vi "이벤트 키 입력 예제.vi"() -> ()   [LabVIEW 2025]
panel:
  out "Boolean":bool
  out "key":string
  in  "stop":bool
  out "count":i32
  # "실행하면 키 입력값을 받고 엔터를 누르면 버튼에 불이 들어오는 구조"
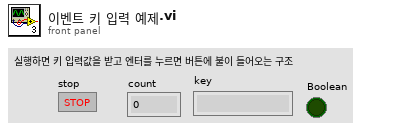
[diagram p1: front panel]
types:
  T1 = typedef "eventvkey.ctl" = enum16{"ASCII", "Enter", "Return", "Shift", "Ctrl", "Alt", "Cmd", "Opt", "Caps", "NumLock", "Clear", "Break", "Up", "Down", "Left", "Right", "Insert", "Delete", "Home", "End", "PageUp", "PageDown", "Escape", "Help", "Pause", "ScrollLock", "F1", "F2", "F3", "F4", "F5", "F6", "F7", "F8", "F9", "F10", "F11", "F12", "F13", "F14", "F15", "F16", "F17", "F18", "F19", "F20", "F21", "F22", "F23", "F24", "Play", "VolumeUp", "VolumeDown", "Mute", "Two Byte Char"}
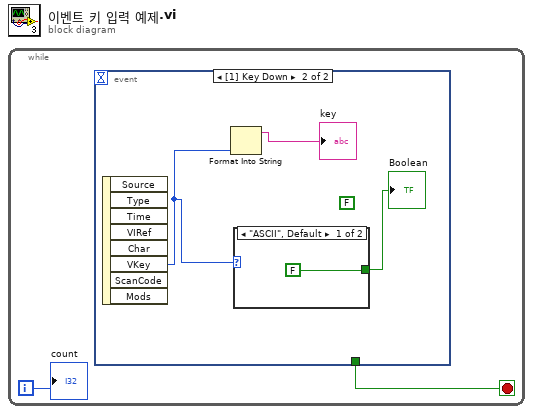
[diagram p0: block diagram]
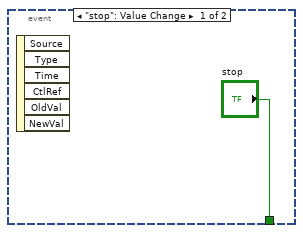
[diagram p2: hidden frame]
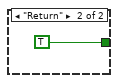
[diagram p3: hidden frame]
diagram:
  n1 = while {
    i -> [w2]
    stop <- w1 stop-if-true
    n2 = event shown="[1] Key Down" {
      selector: _ -> [_ _]
      dyn-events: _ -> [_ _]
      timeout: _ -> [_ _]
      tunnel: ["stop" _] -> w1
      event "stop": Value Change {
        n3 = event-data() -> ()  [unwired: 1 in, 6 out]
      }
      event Key Down {
        (unwired) FALSE
        n4 = event-data() -> ("VKey"=w5:T1)  [unwired: 1 in, 7 out]
        n5 = Format Into String(w5) -> (resulting string=→"key":string)  [unwired: 3 in, 1 out]
        n6 = case shown="\"ASCII\", Default" w5 {
          tunnel: [FALSE TRUE] -> w4
          frame "ASCII", Default {
          }
          frame "Return" {
          }
        }
        "Boolean" <- w4
      }
    }
    "count" <- w2
  }
